vi "To ISO8601 String.vi"(5 "Format Config":T1={"Format"=enum."Extended", "Precision"=enum."Second"}, 7 "Now for Unset? (T)":bool=TRUE, 11 "Time Stamp":timestamp) -> (3 "ISO 8601 UTC":string)   [LabVIEW 2020, in "CDM-Config.lvlib"]
doc: "Converts a LabVIEW timestamp (or Now if not specified) into an ISO-8601 formatted string in the UTC time zone. This is the standard format used for converting LabVIEW Timestamps into strings with this config library.\n\nFormat Config:\n<b>Format</b> - Whether the generated string contains the dashes in the date portion and colon ':' in the time portion or not. The Basic format is suitable for use in filenames.\n\n<b>Precision</b> - How much of the string to generate based on the desired precision needed. \"Day\" excludes the time portion of the string to just specify a date."
uses:
  CDM-Config.lvlib
  Format Config.ctl
  Format.ctl
  Precision.ctl
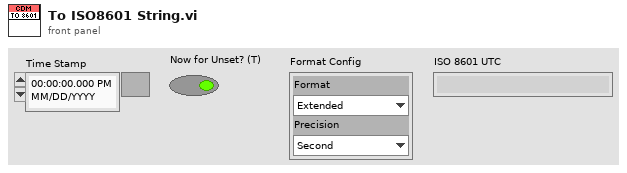
[diagram p1: front panel]
types:
  T1 = typedef "CDM-Config.lvlib/Format Config.ctl" = cluster{"Format":T2, "Precision":T3}
  T2 = typedef "CDM-Config.lvlib/Format.ctl" = enum16{"Extended", "Basic"}
  T3 = typedef "CDM-Config.lvlib/Precision.ctl" = enum16{"Millisecond", "Second", "Minute", "Hour", "Day"}
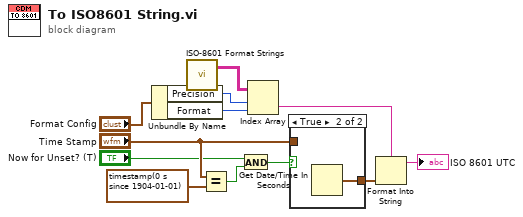
[diagram p0: block diagram]
diagram:
  n1 = Unbundle By Name("Format Config") -> ("Precision"=w6:T3, "Format"=w5:T2)
  n2 = call "ISO-8601 Format Strings.vi"() -> ("Formats"=w4:string[][])  [unwired: 3 in]
  n3 = Equal?(x="Time Stamp", y=timestamp(0 s since 1904-01-01)) -> (x = y?=w9:bool)
  n4 = And(x="Now for Unset? (T)", y=w9) -> (x .and. y?=w8:bool)
  n5 = Index Array(array=w4, index (row)=w6, index (col)=w5) -> (element=w3:string)
  n6 = case shown="True" w8 {
    tunnel: "Time Stamp" -> [w13 _]
    tunnel: [w13 w14] -> w1
    frame False {
    }
    frame True {
      n7 = Get Date/Time In Seconds() -> (seconds since 1Jan1904=w14:timestamp)
    }
  }
  n8 = Format Into String(format string=w3, w1) -> (resulting string=→"ISO 8601 UTC":string)  [unwired: 2 in, 1 out]
